vi "Subscribe.vi"(8 "error in (no error)":errorcluster, 9 "Protocol":T1, 10 "Endpoint":string, 11 "Topic in":refnum<class "Topic.lvclass">) -> (0 "error out":errorcluster, 2 "Subscription":refnum<class "Subscription.lvclass">, 3 "Topic out":refnum<class "Topic.lvclass">)   [LabVIEW 2015, in "NI_AWS_SNS.lvlib" / "Topic.lvclass"]
doc: "Prepares to subscribe an endpoint by sending the endpoint a confirmation message. To actually create a subscription, the endpoint owner must call the Confirm Subscription action with the token from the confirmation message. Confirmation tokens are valid for three days.\n\nThis action is throttled at 100 transactions per second (TPS)."
uses:
  Topic.lvclass
  Subscription/Subscription Protocol.ctl
  Subscription/Subscription.lvclass
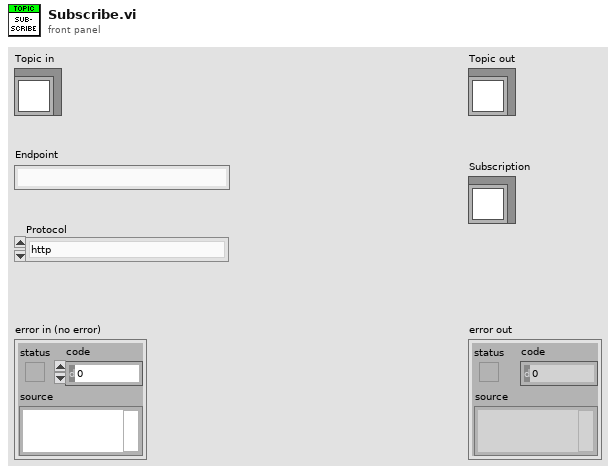
[diagram p1: front panel]
types:
  T1 = typedef "NI_AWS_SNS.lvlib/Subscription.lvclass/Subscription Protocol.ctl" = enum16{"http", "https", "email", "email-json", "sms", "sqs", "application", "lambda"}
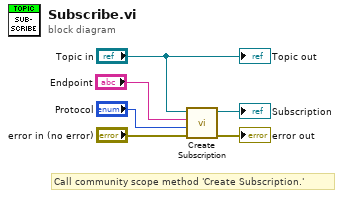
[diagram p0: block diagram]
diagram:
  # "Call community scope method 'Create Subscription.'"
  n1 = call "Create Subscription.vi"("error in (no error)"="error in (no error)", "Protocol"="Protocol", "Endpoint"="Endpoint", "Topic"="Topic in") -> ("error out"=→"error out":errorcluster, "Subscription out"=→"Subscription":refnum<class "Subscription.lvclass">)  [unwired: 6 in]
  "Topic out" <- "Topic in"
